vi "Get_Arguments.vi"(8 "error in (no error)":errorcluster caption="entrée d'erreur (pas d'erreur)", 11 "Flash_Jlink en entrée":refnum<class "Flash_Epox.lvclass">) -> (0 "error out":errorcluster caption="sortie d'erreur", 2 "Arguments":string, 3 "Flash_Jlink en sortie":refnum<class "Flash_Epox.lvclass">)   [LabVIEW 2020, in "Library Test.lvlib" / "Flash_Epox.lvclass"]
uses:
  Flash_Epox.lvclass
  Flash_Epox.lvclass/Flash_Epox.ctl
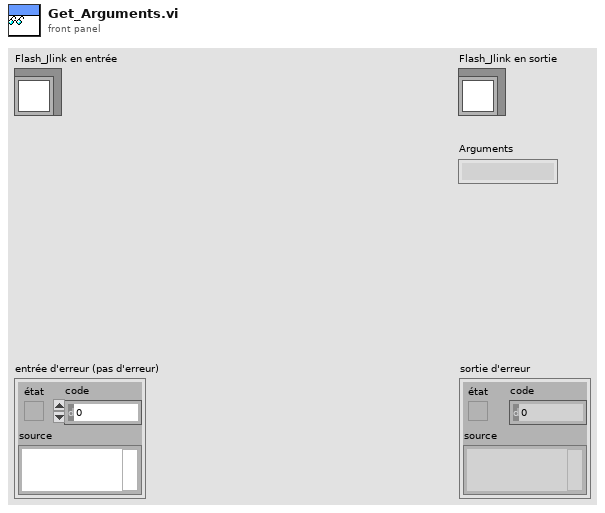
[diagram p1: front panel]
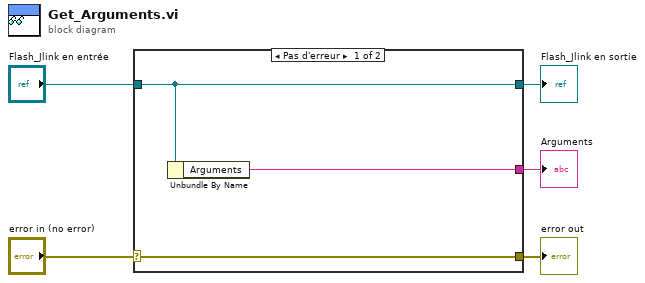
[diagram p0: block diagram]
diagram:
  n1 = case shown="Pas d'erreur" "error in (no error)" {
    selector: "error in (no error)" -> [w8 w9]
    tunnel: [w8 w9] -> w4
    tunnel: [w7 w10] -> w2
    tunnel: "Flash_Jlink en entrée" -> [w7 w10]
    tunnel: [w6 _] -> w1
    frame No Error {
      n2 = Unbundle By Name(w7) -> ("Arguments"=w6:string)
    }
    frame Error {
    }
  }
  "error out" <- w4
  "Flash_Jlink en sortie" <- w2
  "Arguments" <- w1
